vi "Write Raw Data.vi"(8 "error in (no error)":errorcluster, 10 "Raw Data":waveform(dbl), 11 "Diode I-V in":refnum<class "Diode IV.lvclass">) -> (0 "error out":errorcluster, 3 "Diode I-V out":refnum<class "Diode IV.lvclass">)   [LabVIEW 2013, in "Diode Characterization.lvlib" / "Diode IV.lvclass"]
uses:
  Diode IV.lvclass
  Diode IV.lvclass/Diode IV.ctl
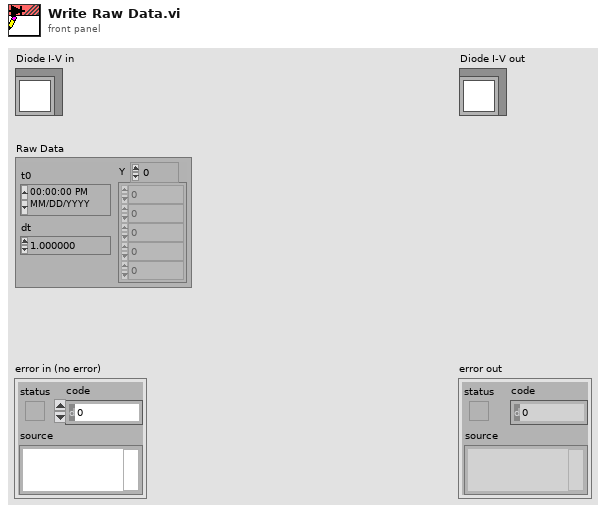
[diagram p1: front panel]
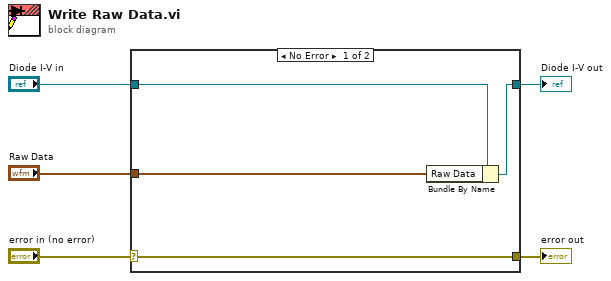
[diagram p0: block diagram]
diagram:
  n1 = case shown="No Error" "error in (no error)" {
    selector: "error in (no error)" -> [w9 w10]
    tunnel: [w9 w10] -> w4
    tunnel: [w7 w11] -> w2
    tunnel: "Diode I-V in" -> [w8 w11]
    tunnel: "Raw Data" -> [w6 _]
    frame No Error {
      n2 = Bundle By Name(cluster=w8, "Raw Data"=w6) -> (w7:refnum<class "Diode IV.lvclass">)
    }
    frame Error {
    }
  }
  "error out" <- w4
  "Diode I-V out" <- w2
